vi "debugMsg.vi"(0 "error in (no error)":errorcluster, 1 "ptr":i64) -> (2 "error out":errorcluster, 3 "ptr out":i64, 4 "msg 2":sgl[](array[numeric]))   [LabVIEW 2016, in "CNet.lvlib"]
uses:
  CNet.lvlib
  Users/jg754/Documents/Visual Studio 2015/Projects/CLearn/x64/Debug/CLearn.dll
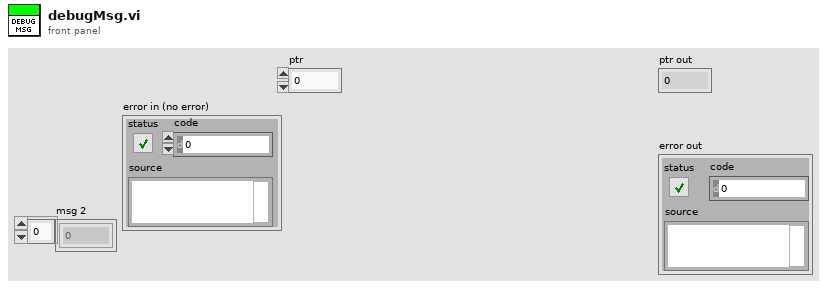
[diagram p1: front panel]
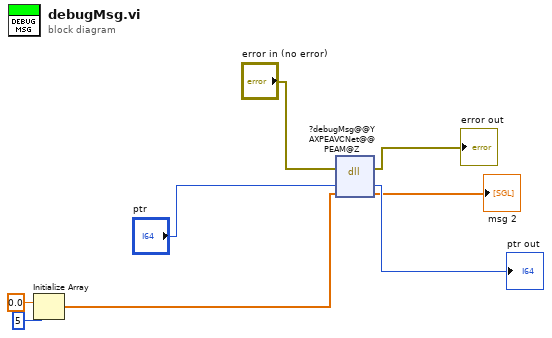
[diagram p0: block diagram]
diagram:
  n1 = Initialize Array(sgl 0.0 ("element"), 5 ("dimension size")) -> (w1:sgl[])
  n2 = dll-call lib="C:/Users/jg754/Documents/Visual Studio 2015/Projects/CLearn/x64/Debug/CLearn.dll" fn="?debugMsg@@YAXPEAVCNet@@PEAM@Z"(error in="error in (no error)", "ptr"="ptr", "msg"=w1) -> (error out=→"error out":errorcluster, "ptr"=→"ptr out":i64, "msg"=→"msg 2":sgl[])  [unwired: 3 in, 1 out]
